vi "DAQ.Write AO.vi"(8 "error in (no error)":errorcluster, 10 "AO []":waveform(dbl)[](array[waveform]), 11 "Instrument.DAQ in":refnum<class "Instrument.DAQ.lvclass">) -> (0 "error out":errorcluster, 2 "AO out []":waveform(dbl)[](array[waveform]), 3 "Instrument.DAQ out":refnum<class "Instrument.DAQ.lvclass">)   [LabVIEW 2019, in "Instrument.Lockin.lvlib" / "Instrument.DAQ.lvclass"]
uses:
  Instrument.DAQ.lvclass
  Instrument.DAQ.lvclass/Instrument.DAQ.ctl
  DAQmx/DAQmx.lvclass
  Generator/Generator.lvclass
panel:
  in  "show graph":bool
  out "Waveform Graph":waveform(dbl)[](graph)
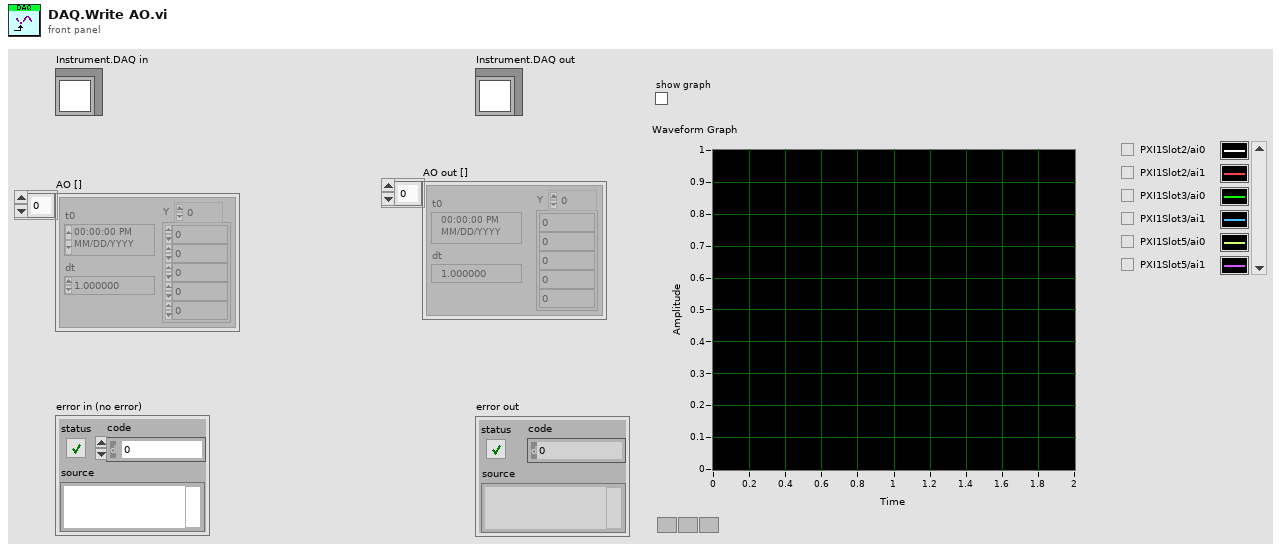
[diagram p1: front panel]
types:
  T1 = typedef "Instrument.Lockin.lvlib/Instrument.DAQ.lvclass/AO.Channel--Cluster--Array.ctl" = T2[]
  T2 = typedef "Instrument.Lockin.lvlib/Instrument.DAQ.lvclass/AO.Channel--Cluster.ctl" = cluster{"Enable?":bool, "Channel":i32, "Amplitude":dbl, "Offset":dbl, "Frequency":dbl, "Phase":dbl, "Function":T3, "Sweeping?":bool, "Limit AC":bool, "Limit DC?":bool, "Duty Cycle":bool}
  T3 = typedef "Instrument.Lockin.lvlib/Instrument.DAQ.lvclass/AO.Channel.Function--Enum.ctl" = enum16{"sine", "square", "triangle", "saw"}
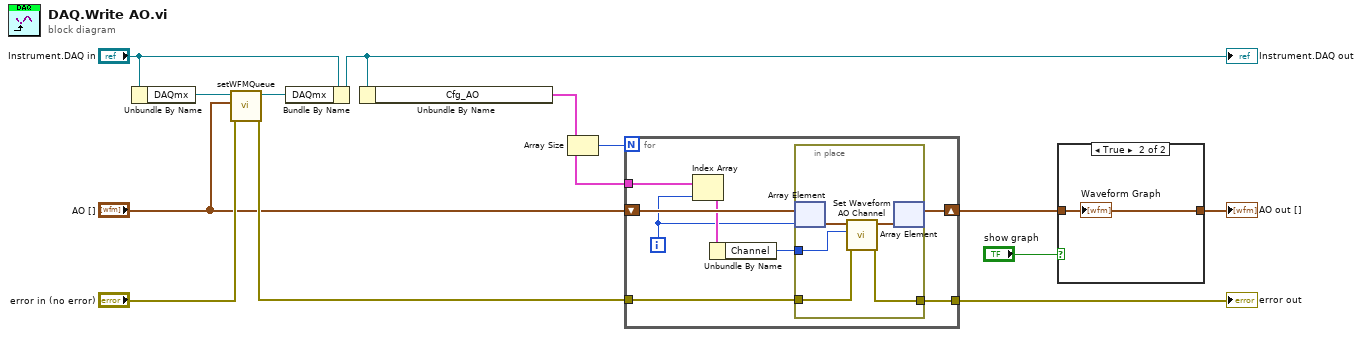
[diagram p0: block diagram]
diagram:
  n1 = Unbundle By Name("Instrument.DAQ in") -> ("DAQmx"=w5:refnum<class "DAQmx.lvclass">)
  n2 = call "setWFMQueue.vi"("error in (no error)"="error in (no error)", "AO"="AO []", "DAQmx in"=w5) -> ("error out"=w2:errorcluster, "DAQmx out"=w4:refnum<class "DAQmx.lvclass">)  [unwired: 7 in]
  n3 = Bundle By Name(cluster="Instrument.DAQ in", "DAQmx"=w4) -> (w9:refnum<class "Instrument.DAQ.lvclass">)
  "Instrument.DAQ out" <- w9
  n4 = Unbundle By Name(w9) -> ("Cfg_AO"=w12:T1)
  n5 = Array Size(array=w12) -> (size(s)=w13:i32)
  n6 = for {
    N: w13 -> [_]
    tunnel: w2 -> [w20]
    tunnel: [w19] -> w8
    shift-right: [w18] -> w7
    shift-left: "AO []" -> [w21]
    tunnel: w12 -> [w17]
    i -> [w14]
    n7 = Index Array(array=w17, index=w14) -> (element=w16:T2)
    n8 = Unbundle By Name(w16) -> ("Channel"=w15:i32)
    n9 = in-place {
      in-place-border: w20 -> [w24]
      in-place-border: [w23] -> w19
      in-place-border: w15 -> [w22]
      n10 = in-place-array #1(w21, w14) -> (w26:waveform(dbl))
      n11 = call "Set Waveform AO Channel.vi"("error in (no error)"=w24, "AO Channel"=w22, "Waveform in"=w26) -> ("error out"=w23:errorcluster, "Waveform out"=w25:waveform(dbl))  [unwired: 7 in]
      n12 = in-place-array #1(w25) -> (w18:waveform(dbl)[])  [unwired: 1 out]
    }
  }
  "error out" <- w8
  n13 = case shown="True" "show graph" {
    tunnel: w7 -> [w27 w28]
    tunnel: [w27 w28] -> w6
    frame False {
    }
    frame True {
      "Waveform Graph" <- w28
    }
  }
  "AO out []" <- w6
